vi "Setup and start acquisition.vi"(8 "error in (no error)":errorcluster, 9 "Final Angle P1":dbl, 10 "FCR Mod ID":i32, 11 "DAQ Mod ID":i32) -> (0 "error out":errorcluster)   [LabVIEW 2020]
uses:
  Newport_FCR100/Libraries/FCR100/Support/Device state -- enum.ctl
  NI_DAQ/Libraries/NI DAQ/Support/Task list.ctl
  Newport_FCR100/Libraries/FCR100/FCR100.lvlib
  NI_DAQ/Libraries/NI DAQ/NI DAQ.lvlib
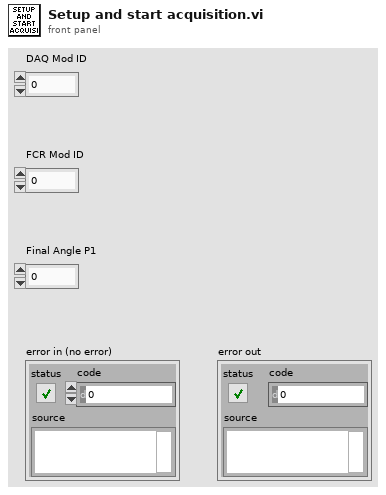
[diagram p1: front panel]
types:
  T1 = typedef "NI DAQ.lvlib/Task list.ctl" = enum16{"All", "DO task", "DI task", "AO task", "AI task"}
  T2 = typedef "FCR100.lvlib/Device state -- enum.ctl" = enum16{"Not referenced", "Configuration", "Disable", "Ready", "Homing", "Motion"}
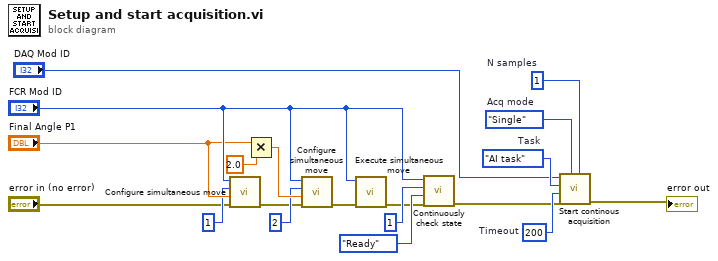
[diagram p0: block diagram]
diagram:
  w4 = 1  # N samples
  w5 = enum16{"Single", "Multiple"}."Single"  # Acq mode
  w6 = 200  # Timeout
  w7 = Task_list."AI task"  # Task
  n1 = call "Configure simultaneous move.vi"("error in"="error in (no error)", "Position"="Final Angle P1", "Address"=u8 1, "Module ID"="FCR Mod ID") -> ("error out"=w10:errorcluster)  [unwired: 7 in]
  n2 = Multiply(x="Final Angle P1", y=2.0) -> (x*y=w14:dbl)
  n3 = call "Configure simultaneous move.vi"("error in"=w10, "Position"=w14, "Address"=u8 2, "Module ID"="FCR Mod ID") -> ("error out"=w15:errorcluster)  [unwired: 7 in]
  n4 = call "Execute simultaneous move.vi"("error in"=w15, "Module ID"="FCR Mod ID") -> ("error out"=w16:errorcluster)  [unwired: 9 in]
  n5 = call "Continuously check state.vi"("error in"=w16, "Desired state"=Device_state_--_enum."Ready", "Address"=u8 1, "Module ID"="FCR Mod ID") -> ("error out"=w3:errorcluster)  [unwired: 7 in]
  n6 = call "Start continous acquisition.vi"("N samples"=w4, "Samples"=w5, "error in"=w3, "Timeout"=w6, "Task list"=w7, "Module ID"="DAQ Mod ID") -> ("error out"=→"error out":errorcluster)  [unwired: 5 in]
